vi "_Clear Array - FP.vi"(0 "GObject in":refnum<vi>, 5 "error in (no error)":errorcluster) -> (14 "changed?":bool, 19 "error out":errorcluster)   [LabVIEW 2015, in "QD_Erease Data.lvlib"]
uses:
  QD_Erease Data.lvlib
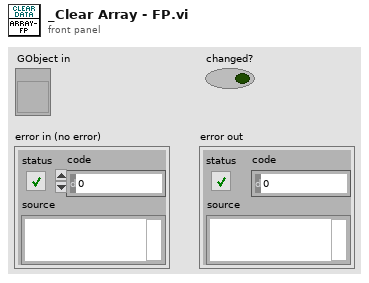
[diagram p1: front panel]
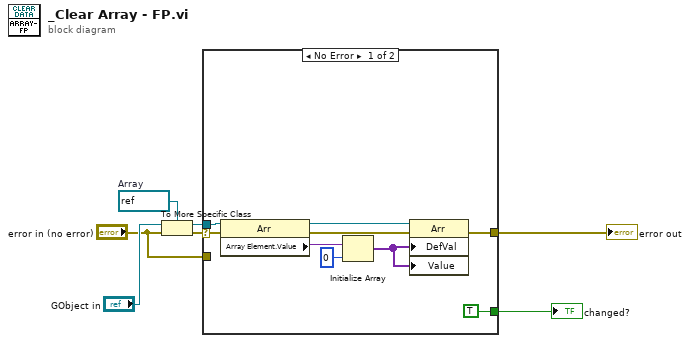
[diagram p0: block diagram]
diagram:
  w6 = refnum<vi> refnum  # Array
  n1 = To More Specific Class(target class=w6, reference="GObject in", error in="error in (no error)") -> (specific class reference=w2:refnum<vi>, error out=w3:errorcluster)
  n2 = case shown="No Error" w3 {
    selector: w3 -> [w11 _]
    tunnel: [w10 w17] -> w1
    tunnel: w2 -> [w12 _]
    tunnel: "error in (no error)" -> [_ w17]
    tunnel: [TRUE _] -> w7
    frame No Error {
      n3 = property class="Arr"(reference=w12, error in=w11) -> (reference out=w15:refnum<vi>, error out=w16:errorcluster, "Array Element.Value"=w14:variant)
      n4 = Initialize Array(w14, 0 ("dimension size")) -> (w9:variant[])
      n5 = property class="Arr"(reference=w15, error in=w16, "DefVal"=w9, "Value"=w9) -> (error out=w10:errorcluster)  [unwired: 1 out]
    }
    frame Error {
    }
  }
  "changed?" <- w7
  "error out" <- w1
